vi "Limelight_Calculation.vi"() -> (1 "driveCommand":dbl(knob)=-0.0 scale=0.0..1.0, 2 "steerCommand":dbl(knob)=nan scale=-1.0..1.0)   [LabVIEW 2019]
uses:
  <vilib>/Rock Robotics/Network Tables/NT Read Number.vi
panel:
  out "targetValid":bool
  out "output cluster":T1
  in  "maxDrive":dbl(slide)=0.6824817518248175 min=0.0 max=1.0 step=0.01 scale=0.0..1.0
  in  "driveK":dbl(slide)=0.26277372262773724 min=0.0 max=1.0 step=0.05 scale=0.0..1.0
  in  "limelightGoalArea":dbl(slide)=14.872262773722628 min=0.1 max=25.0 step=0.25 scale=0.0..25.0
  in  "aimDeadband":dbl min=0.0 max=10.0 step=0.25
  in  "minSteerCommand":dbl(slide)=0.2717391304347826 min=0.0 max=0.5 step=0.05 scale=0.0..0.5
  in  "steeringK":dbl(slide)=0.025362318840579712 min=0.0 max=0.25 step=0.01 scale=0.0..0.25
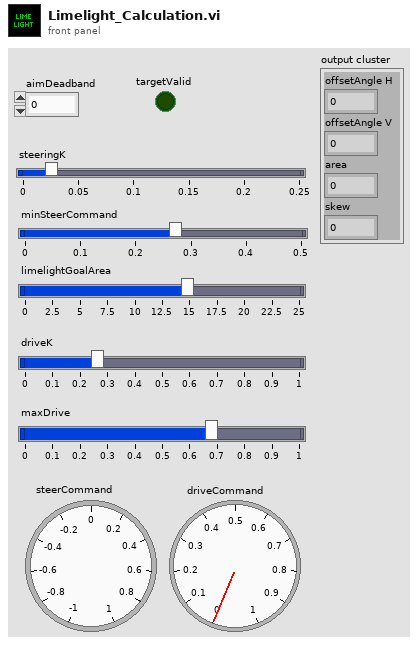
[diagram p1: front panel]
types:
  T1 = cluster{"offsetAngle H":dbl, "offsetAngle V":dbl, "area":dbl, "skew":dbl}
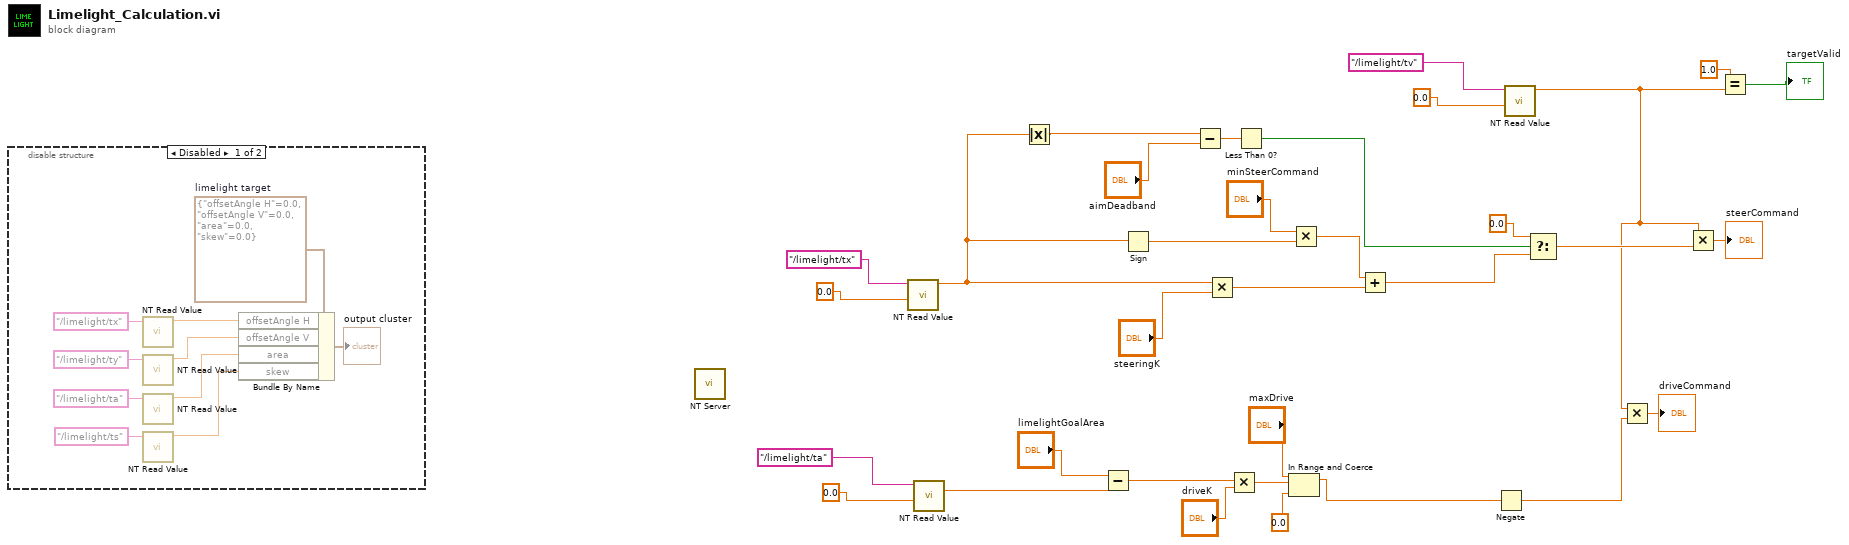
[diagram p0: block diagram]
diagram:
  n1 = disable-structure shown="Disabled" {
    frame Disabled {
      w39 = T1 {"offsetAngle H"=0.0, "offsetAngle V"=0.0, "area"=0.0, "skew"=0.0}  # limelight target
      n2 = call-poly <vilib>:"NT Read Value.vi"("Name"="/limelight/tx") -> ("Numeric"=w38:dbl)  [unwired: 9 in, 1 out]
      n3 = call-poly <vilib>:"NT Read Value.vi"("Name"="/limelight/ty") -> ("Numeric"=w37:dbl)  [unwired: 9 in, 1 out]
      n4 = call-poly <vilib>:"NT Read Value.vi"("Name"="/limelight/ta") -> ("Numeric"=w36:dbl)  [unwired: 9 in, 1 out]
      n5 = call-poly <vilib>:"NT Read Value.vi"("Name"="/limelight/ts") -> ("Numeric"=w35:dbl)  [unwired: 9 in, 1 out]
      n6 = Bundle By Name(cluster=w39, "offsetAngle H"=w38, "offsetAngle V"=w37, "area"=w36, "skew"=w35) -> (→"output cluster":T1)
    }
    frame Enabled {
    }
  }
  n7 = call <vilib>:"NT Server.vi"() -> ()  [unwired: 12 in]
  n8 = call-poly <vilib>:"NT Read Value.vi"("Default Value"=0.0, "Name"="/limelight/tx") -> ("Numeric"=w6:dbl)  [unwired: 8 in, 1 out]
  n9 = call-poly <vilib>:"NT Read Value.vi"("Default Value"=0.0, "Name"="/limelight/ta") -> ("Numeric"=w15:dbl)  [unwired: 8 in, 1 out]
  n10 = Absolute Value(x=w6) -> (abs(x)=w29:dbl)
  n11 = Subtract(x="limelightGoalArea", y=w15) -> (x-y=w13:dbl)
  n12 = Sign(1:w6) -> (0:w17:dbl)
  n13 = Subtract(x=w29, y="aimDeadband") -> (x-y=w31:dbl)
  n14 = Multiply(x=w6, y="steeringK") -> (x*y=w26:dbl)
  n15 = Multiply(x=w13, y="driveK") -> (x*y=w12:dbl)
  n16 = Less Than 0?(x=w31) -> (x < 0?=w32:bool)
  n17 = In Range and Coerce(upper limit="maxDrive", x=w12, lower limit=0.0) -> (coerced(x)=w8:dbl)  [unwired: 1 out]
  n18 = Multiply(x="minSteerCommand", y=w17) -> (x*y=w28:dbl)
  n19 = Add(x=w28, y=w26) -> (x+y=w5:dbl)
  n20 = Negate(x=w8) -> (-x=w7:dbl)
  n21 = call-poly <vilib>:"NT Read Value.vi"("Default Value"=0.0, "Name"="/limelight/tv") -> ("Numeric"=w1:dbl)  [unwired: 8 in, 1 out]
  n22 = Select(t=0.0, s=w32, f=w5) -> (s? t:f=w20:dbl)
  n23 = Multiply(x=w1, y=w7) -> (x*y=→"driveCommand":dbl)
  n24 = Multiply(x=w1, y=w20) -> (x*y=→"steerCommand":dbl)
  n25 = Equal?(x=1.0, y=w1) -> (x = y?=→"targetValid":bool)
